vi "전략1.vi"() -> ()   [LabVIEW 2015]
uses:
  <vilib>/NXT/Subs/MotorOutput.ctl
  <vilib>/NXT/Block Support/NXT_InputPort.ctl
  <vilib>/NXT/Dual Mode Library/Sensors/Light_On.vi
  <vilib>/NXT/Dual Mode Library/Sensors/Sonar_cm.vi
  <vilib>/NXT/Dual Mode Library/Motors/MotorReverse.vi
  <vilib>/NXT/Dual Mode Library/Motors/MotorOn.vi
  <vilib>/NXT/Dual Mode Library/Waits/Wait_Num.vi
panel:
  in  "B포트 3":T1=3 items=["Port A", "Port B", "Port C", "All Ports"]
  in  "Power (75) 3":i32=100
  in  "Distance (cm)":i16=50
  in  "Port (Port 4)":T2 items=["Port 1", "Port 2", "Port 3", "Port 4"]
  in  "Time (sec) 2":sgl=0.5
  in  "B포트 2":T1=3 items=["Port A", "Port B", "Port C", "All Ports"]
  in  "Power (75) 2":i32=100
  in  "빛센서":T2=1 items=["Port 1", "Port 2", "Port 3", "Port 4"]
  in  "정지":bool
  in  "Time (sec)":sgl=0.9
  in  "Output Port (All Ports) 3":T1=2 items=["Port A", "Port B", "Port C", "All Ports"]
  in  "전진파워":i32=100
  in  "Output Port (All Ports) 2":T1 items=["Port A", "Port B", "Port C", "All Ports"]
  in  "후진파워":i32=100
  in  "B포트":T1=3 items=["Port A", "Port B", "Port C", "All Ports"]
  in  "Power (75)":i32=100
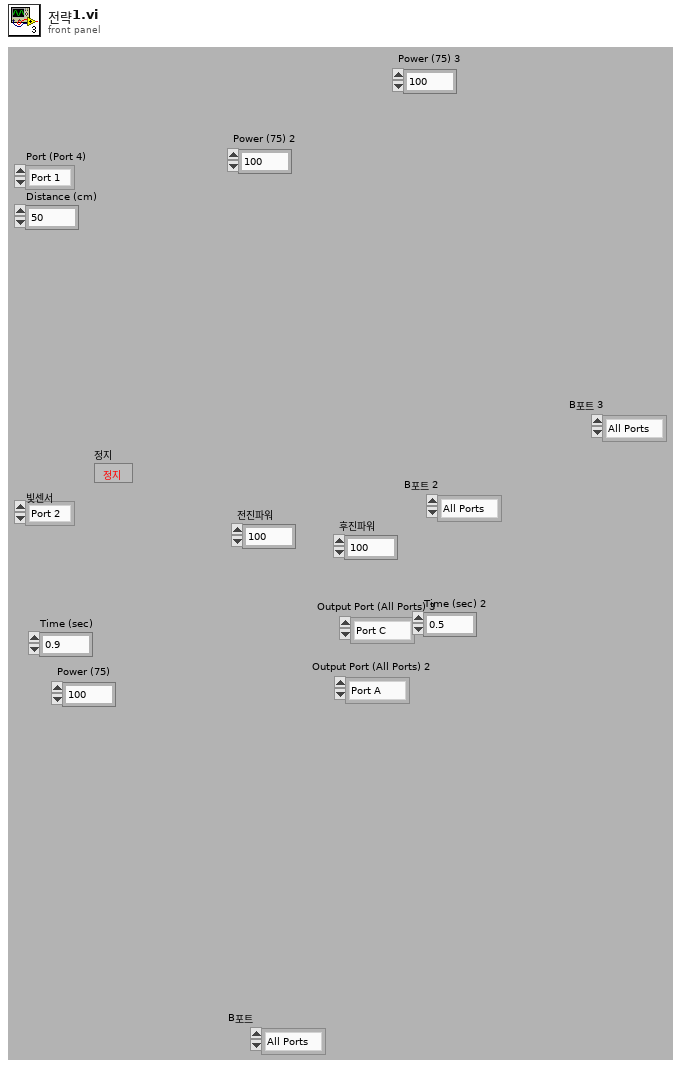
[diagram p1: front panel]
types:
  T1 = typedef "MotorOutput.ctl" = u8
  T2 = typedef "NXT_InputPort.ctl" = u32
  T3 = typedef "LVHSConnector.ctl" = refnum<class "BrickReference.lvclass">
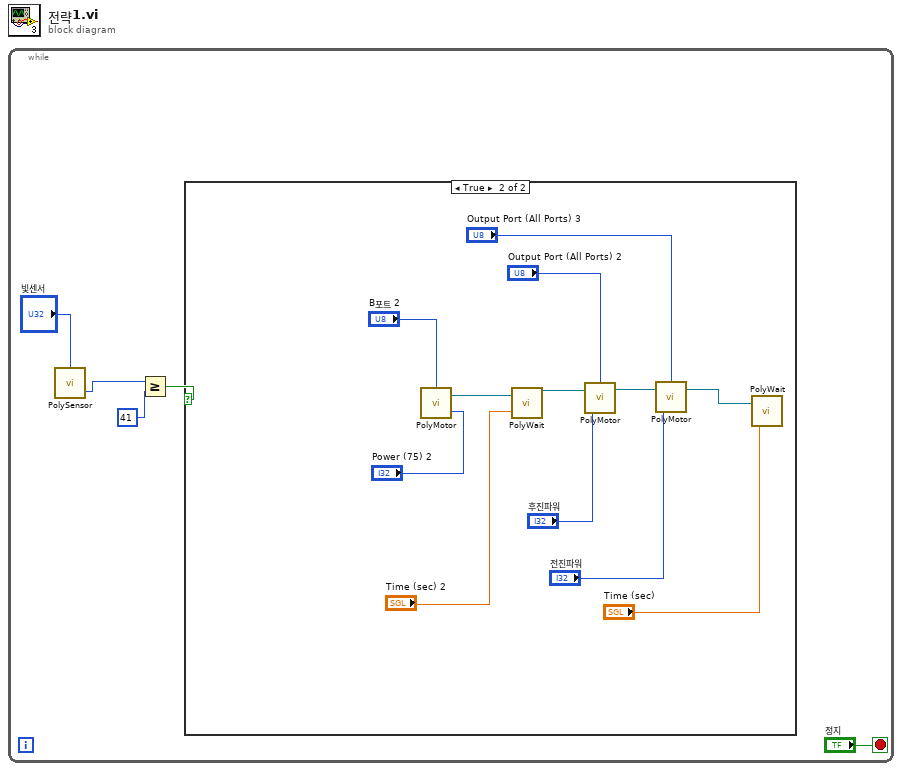
[diagram p0: block diagram]
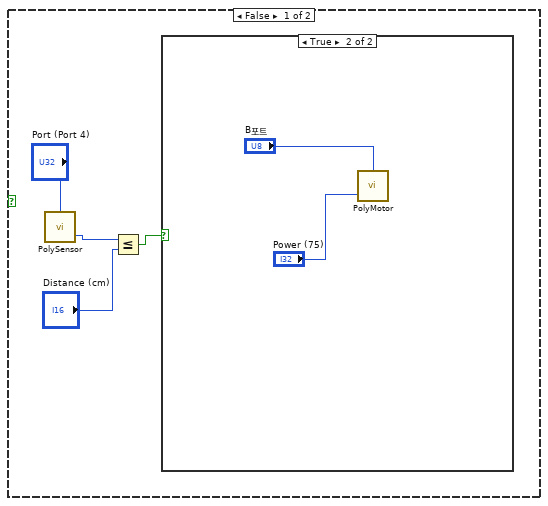
[diagram p2: hidden frame]
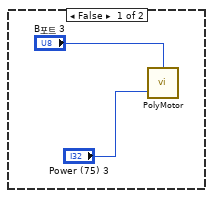
[diagram p3: hidden frame]
diagram:
  n1 = while {
    stop <- "정지" stop-if-true
    n2 = call-poly <vilib>:"PolySensor.vi"("Port (Port 3)"="빛센서") -> ("Scaled Value"=w3:i16)  [unwired: 2 in, 1 out]
    n3 = Greater Or Equal?(x=w3, y=41) -> (x >= y?=w1:bool)
    n4 = case shown="True" w1 {
      frame False {
        n5 = call-poly <vilib>:"PolySensor.vi"("Port (Port 4)"="Port (Port 4)") -> ("Distance (cm)"=w6:i16)  [unwired: 2 in, 1 out]
        n6 = Less Or Equal?(x=w6, y="Distance (cm)") -> (x <= y?=w8:bool)
        n7 = case shown="True" w8 {
          frame False {
            n8 = call-poly <vilib>:"PolyMotor.vi"("Power (75)"="Power (75) 3", "Output Port (All Ports)"="B포트 3") -> ()  [unwired: 2 in, 1 out]
          }
          frame True {
            n9 = call-poly <vilib>:"PolyMotor.vi"("Power (75)"="Power (75)", "Output Port (All Ports)"="B포트") -> ()  [unwired: 2 in, 1 out]
          }
        }
      }
      frame True {
        n10 = call-poly <vilib>:"PolyMotor.vi"("Power (75)"="Power (75) 2", "Output Port (All Ports)"="B포트 2") -> ("NXT/EV3"=w15:T3)  [unwired: 2 in]
        n11 = call-poly <vilib>:"PolyWait.vi"("Time (1 sec)"="Time (sec) 2", "NXT/EV3"=w15) -> ("NXT/EV3"=w14:T3)  [unwired: 2 in]
        n12 = call-poly <vilib>:"PolyMotor.vi"("Power (75)"="후진파워", "NXT/EV3"=w14, "Output Port (All Ports)"="Output Port (All Ports) 2") -> ("NXT/EV3"=w23:T3)  [unwired: 1 in]
        n13 = call-poly <vilib>:"PolyMotor.vi"("Power (75)"="전진파워", "NXT/EV3"=w23, "Output Port (All Ports)"="Output Port (All Ports) 3") -> ("NXT/EV3"=w19:T3)  [unwired: 1 in]
        n14 = call-poly <vilib>:"PolyWait.vi"("Time (1 sec)"="Time (sec)", "NXT/EV3"=w19) -> ()  [unwired: 2 in, 1 out]
      }
    }
  }
